vi "TriggerConfigure.vi"(2 "TriggleSetting":T1={"Type"=enum."Immediate", "Source"="", "Horizontal Position (%)"=2.0, "slope"=10280, "level"=0.0} {"level" format="%0.2f"; "slope" items=["上升"=10280, "下降"=10171]; "Horizontal Position (%)" scale=0.0..1.0}, 3 "Error In":errorcluster caption="error in", 4 "Task In":refnum<k21>) -> (0 "Error Out":errorcluster caption="error out", 1 "Task Out":refnum<k21>)   [LabVIEW 2012]
uses:
  GlobalVariable.vi
  <vilib>/DAQmx/configure/trigger.llb/DAQmx Reference Trigger (Digital Edge).vi
  <vilib>/DAQmx/configure/trigger.llb/DAQmx Reference Trigger (Analog Edge).vi
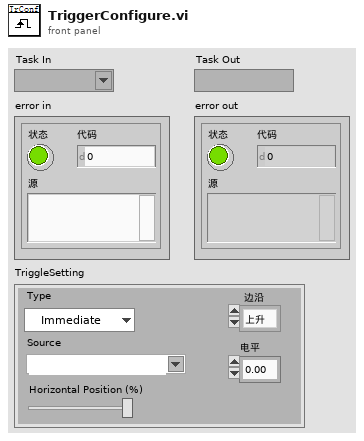
[diagram p1: front panel]
types:
  T1 = cluster{"Type":enum16{"Immediate", "Digital", "Edge"}, "Source":string, "Horizontal Position (%)":dbl, "slope":i32, "level":dbl}
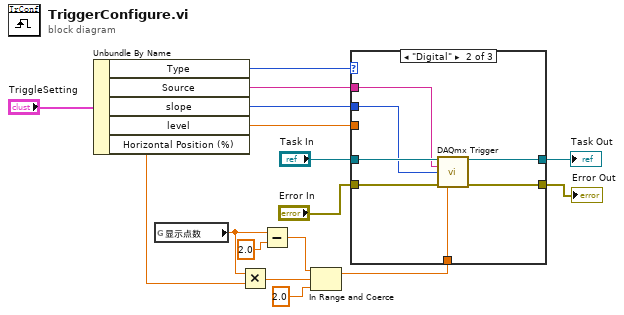
[diagram p0: block diagram]
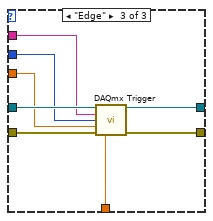
[diagram p3: hidden frame]
diagram:
  n1 = Unbundle By Name("TriggleSetting") -> ("Type"=w5:enum16{"Immediate", "Digital", "Edge"}, "Source"=w11:string, "slope"=w10:i32, "level"=w9:dbl, "Horizontal Position (%)"=w4:dbl)
  n2 = global read "GlobalVariable.vi" "显示点数"() -> (w3:dbl)
  n3 = Multiply(x=w3, y=w4) -> (x*y=w8:dbl)
  n4 = Subtract(x=w3, y=2.0) -> (x-y=w1:dbl)
  n5 = In Range and Coerce(upper limit=w1, x=w8, lower limit=2.0 ("下限")) -> (coerced(x)=w6:dbl)  [unwired: 1 out]
  n6 = case shown="\"Digital\"" w5 {
    tunnel: "Task In" -> [w18 w25 w33]
    tunnel: "Error In" -> [w17 w24 w32]
    tunnel: [w18 w22 w30] -> w14
    tunnel: [w17 w23 w31] -> w13
    tunnel: w11 -> [_ w21 w29]
    tunnel: w6 -> [_ w20 w28]
    tunnel: w10 -> [_ w19 w27]
    tunnel: w9 -> [_ _ w26]
    frame "Immediate", Default {
    }
    frame "Digital" {
      n7 = call-poly <vilib>:"DAQmx Trigger.vi"("task/channels in"=w25, "source"=w21, "edge"=w19, "error in"=w24, "pretrigger samples per channel"=w20) -> ("task out"=w22:refnum<k21>, "error out"=w23:errorcluster)  [unwired: 9 in]
    }
    frame "Edge" {
      n8 = call-poly <vilib>:"DAQmx Trigger.vi"("task/channels in"=w33, "source"=w29, "slope"=w27, "level"=w26, "error in"=w32, "pretrigger samples per channel"=w28) -> ("task out"=w30:refnum<k21>, "error out"=w31:errorcluster)  [unwired: 8 in]
    }
  }
  "Task Out" <- w14
  "Error Out" <- w13
